vi "ELVIS III v1.1 Open AI (Continuous).vi"(4 "Max Value":dbl[](array[numeric]), 6 "Min Value":dbl[](array[numeric]), 8 "error in (no error)":errorcluster, 10 "Channel Names":string[](array[string]), 11 "Resource name":T7 caption="RIO Device") -> (0 "error out":errorcluster, 1 "Bank Count":u8[](array[numeric]), 2 "AI (Continuous) Channels List":T3 caption="AI Continuous Channels List", 3 "AI (Continuous) Ref Out":T5 caption="AI Continuous Ref Out", 5 "AI (Continous) Read Scale Constants List":T1)   [LabVIEW 2021]
uses:
  <vilib>/userDefined/High Color/nirio_resource_hc.ctl
  <vilib>/myRIO/Common/Instrument Driver Framework/Utilities/typedefs/myRIO v1.0 Reference.ctl
  <vilib>/myRIO/Common/Instrument Driver Framework/Utilities/typedefs/Generic FPGA Reference.ctl
  <vilib>/myRIO/Common/Instrument Driver Framework/ELVIS III v1.0/AI Continuous/typedefs/AI Continuous Channels List.ctl
  <vilib>/myRIO/Common/Instrument Driver Framework/ELVIS III v1.0/AI Continuous/typedefs/ELVIS III v1.0 AI Continuous Channels Enum.ctl
  <vilib>/myRIO/Common/Instrument Driver Framework/Utilities/typedefs/Analog Scaling Constants List.ctl
  <vilib>/myRIO/Common/Instrument Driver Framework/Utilities/typedefs/Analog Scaling Constants.ctl
  <vilib>/myRIO/Common/Instrument Driver Framework/myRIO v1.0/AI Continuous/typedefs/AI Continuous Channels Enum.ctl
  <vilib>/myRIO/Common/Instrument Driver Framework/ELVIS III v1.0/AI Continuous/vis/ELVIS III v1.0 Build MUX Configuration AI Continuous.vi
  <vilib>/Utility/VariantDataType/GetNumericInfo.vi
  <vilib>/myRIO/Common/Instrument Driver Framework/ELVIS III v1.0/Resource Manager/vis/ELVIS III v1.0 Reserve Channel List.vi
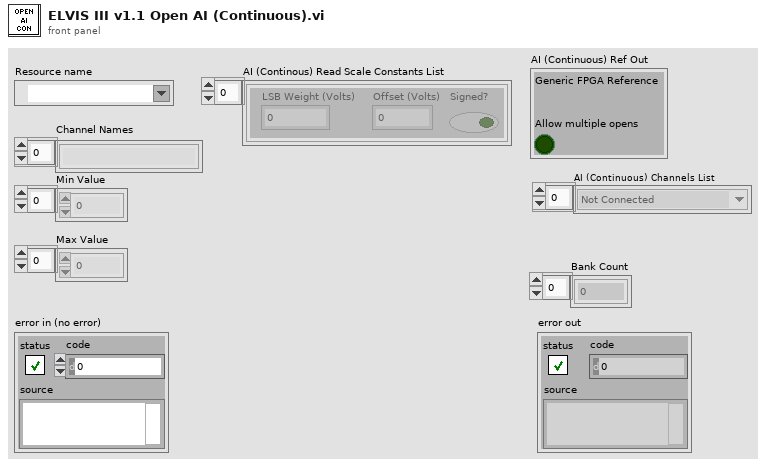
[diagram p1: front panel]
types:
  T1 = typedef "Analog Scaling Constants List.ctl" = T2[]
  T2 = typedef "Analog Scaling Constants.ctl" = cluster{"LSB Weight (Volts)":dbl, "Offset (Volts)":dbl, "Signed?":bool}
  T3 = typedef "AI Continuous Channels List.ctl" = T4[]
  T4 = typedef "ELVIS III v1.0 AI Continuous Channels Enum.ctl" = enum16{"Not Connected", "A/AI0 (Continuous)", "A/AI1 (Continuous)", "A/AI2 (Continuous)", "A/AI3 (Continuous)", "A/AI4 (Continuous)", "A/AI5 (Continuous)", "A/AI6 (Continuous)", "A/AI7 (Continuous)", "A/AI0 (DIFF Continuous)", "A/AI1 (DIFF Continuous)", "A/AI2 (DIFF Continuous)", "A/AI3 (DIFF Continuous)", "B/AI0 (Continuous)", "B/AI1 (Continuous)", "B/AI2 (Continuous)", "B/AI3 (Continuous)", "B/AI4 (Continuous)", "B/AI5 (Continuous)", "B/AI6 (Continuous)", "B/AI7 (Continuous)", "B/AI0 (DIFF Continuous)", "B/AI1 (DIFF Continuous)", "B/AI2 (DIFF Continuous)", "B/AI3 (DIFF Continuous)"}
  T5 = typedef "myRIO v1.0 Reference.ctl" = cluster{"Generic FPGA Reference":T6, "Allow multiple opens":bool}
  T6 = typedef "Generic FPGA Reference.ctl" = refnum<k20>
  T7 = typedef "nirio_resource_hc.ctl" = tag
  T8 = typedef "AI Continuous Channels Enum.ctl" = enum16{"Not Connected", "A/AI0 (Continuous)", "A/AI1 (Continuous)", "A/AI2 (Continuous)", "A/AI3 (Continuous)", "A/AI4 (Continuous)", "A/AI5 (Continuous)", "A/AI6 (Continuous)", "A/AI7 (Continuous)", "A/AI0 (DIFF Continuous)", "A/AI1 (DIFF Continuous)", "A/AI2 (DIFF Continuous)", "A/AI3 (DIFF Continuous)", "B/AI0 (Continuous)", "B/AI1 (Continuous)", "B/AI2 (Continuous)", "B/AI3 (Continuous)", "B/AI4 (Continuous)", "B/AI5 (Continuous)", "B/AI6 (Continuous)", "B/AI7 (Continuous)", "B/AI0 (DIFF Continuous)", "B/AI1 (DIFF Continuous)", "B/AI2 (DIFF Continuous)", "B/AI3 (DIFF Continuous)"}
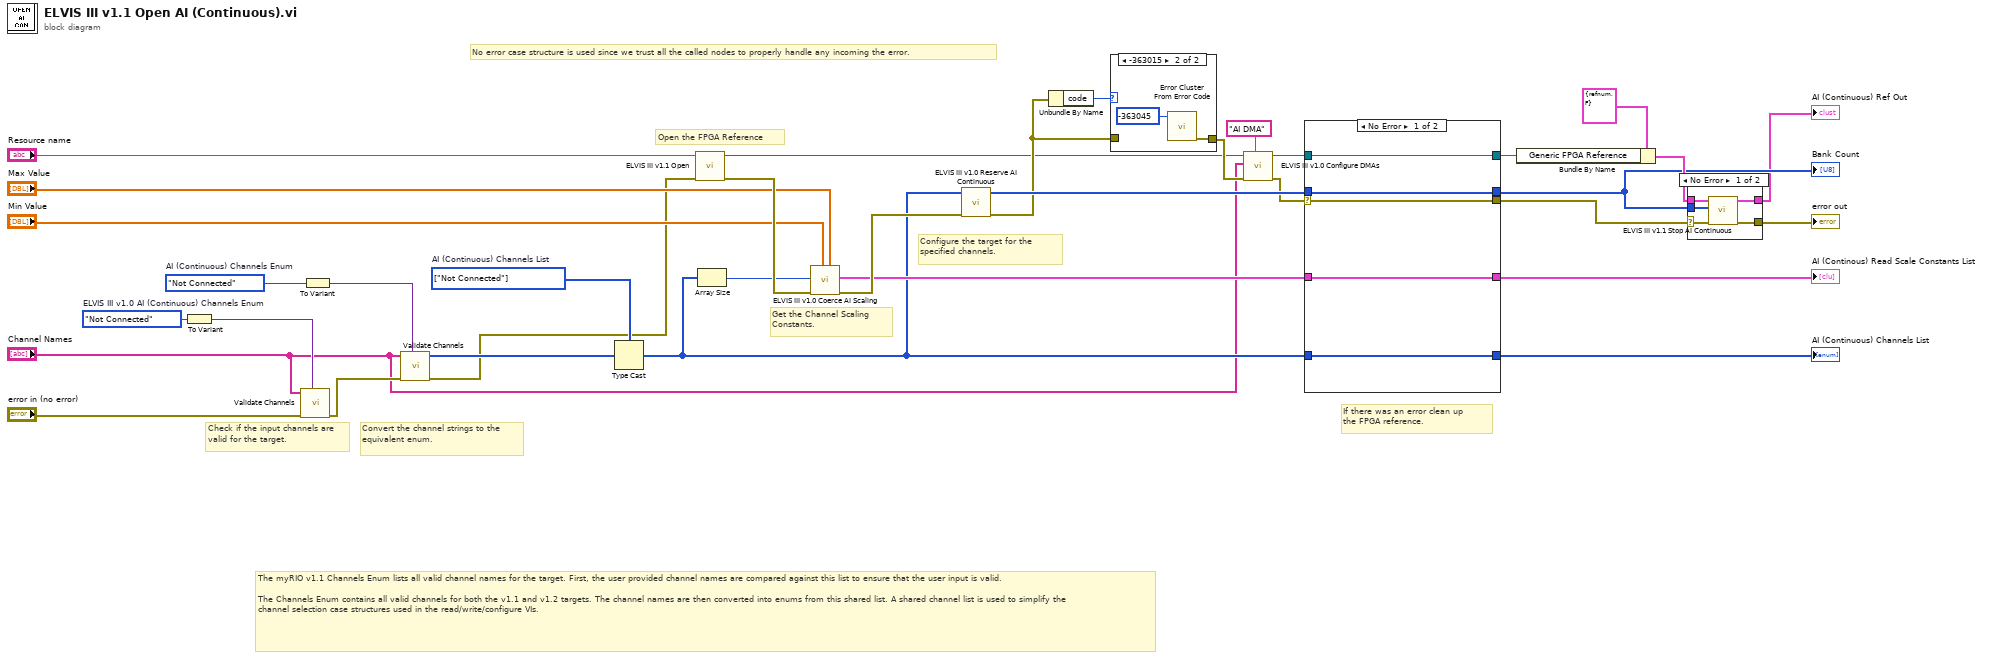
[diagram p0: block diagram]
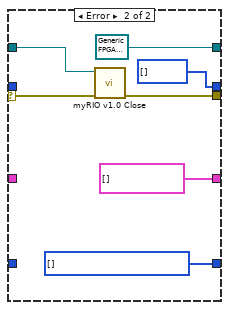
[diagram p4: hidden frame]
diagram:
  w20 = AI_Continuous_Channels_Enum."Not Connected"  # AI (Continuous) Channels Enum
  w25 = T3 [enum."Not Connected"] items=["Not Connected", "A/AI0 (Continuous)", "A/AI1 (Continuous)", "A/AI2 (Continuous)", "A/AI3 (Continuous)", "A/AI4 (Continuous)", "A/AI5 (Continuous)", "A/AI6 (Continuous)", "A/AI7 (Continuous)", "A/AI0 (DIFF Continuous)", "A/AI1 (DIFF Continuous)", "A/AI2 (DIFF Continuous)", "A/AI3 (DIFF Continuous)", "B/AI0 (Continuous)", "B/AI1 (Continuous)", "B/AI2 (Continuous)", "B/AI3 (Continuous)", "B/AI4 (Continuous)", "B/AI5 (Continuous)", "B/AI6 (Continuous)", "B/AI7 (Continuous)", "B/AI0 (DIFF Continuous)", "B/AI1 (DIFF Continuous)", "B/AI2 (DIFF Continuous)", "B/AI3 (DIFF Continuous)"]  # AI (Continuous) Channels List
  w26 = ELVIS_III_v1.0_AI_Continuous_Channels_Enum."Not Connected"  # ELVIS III v1.0 AI (Continuous) Channels Enum
  # "Get the Channel Scaling Constants."
  # "The myRIO v1.1 Channels Enum lists all valid channel names for the target. First, the user provided channel names are compared against this list to ensure that the user input is valid.\n\nThe Channels Enum contains all valid channels for both the v1.1 and v1.2 targets. The channel names are then converted into enums from this shared list. A shared channel list is used to simplify the channel selection case structures used in the read/write/configure VIs."
  # "If there was an error clean up the FPGA reference."
  # "Configure the target for the specified channels."
  # "Open the FPGA Reference"
  # "No error case structure is used since we trust all the called nodes to properly handle any incoming the error."
  # "Convert the channel strings to the equivalent enum."
  # "Check if the input channels are valid for the target."
  n1 = To Variant(anything=w26) -> (Variant=w33:variant)
  n2 = call <vilib>:"Validate Channels.vi"("Channels Enum Variant"=w33, "error in (no error)"="error in (no error)", "Channel Names"="Channel Names") -> ("error out"=w17:errorcluster)  [unwired: 7 in, 1 out]
  n3 = To Variant(anything=w20) -> (Variant=w19:variant)
  n4 = call <vilib>:"Validate Channels.vi"("Channels Enum Variant"=w19, "error in (no error)"=w17, "Channel Names"="Channel Names") -> ("error out"=w16:errorcluster, "Index Array"=w18:u16[])  [unwired: 7 in]
  n5 = Type Cast(type=w25, x=w18) -> (*(type *) &x=w15:T3)
  n6 = call <vilib>:"ELVIS III v1.1 Open.vi"("error in (no error)"=w16, "Resource name"="Resource name") -> ("error out"=w32:errorcluster, "myRIO FPGA Ref Out"=w10:T6)  [unwired: 8 in]
  n7 = Array Size(array=w15) -> (size(s)=w30:i32)
  n8 = call <vilib>:"ELVIS III v1.0 Coerce AI Scaling.vi"("Max Value"="Max Value", "Min Value"="Min Value", "error in (no error)"=w32, "Channel List Size"=w30) -> ("error out"=w31:errorcluster, "Scale Constants Array"=w29:T1)  [unwired: 6 in]
  n9 = call <vilib>:"ELVIS III v1.0 Reserve AI Continuous.vi"("error in (no error)"=w31, "AI (Continuous) Channels List"=w15) -> ("error out"=w12:errorcluster, "Bank Count"=w14:u8[])  [unwired: 8 in]
  n10 = Unbundle By Name(w12) -> ("code"=w13:i32)
  n11 = case shown="-363015" w13 {
    tunnel: w12 -> [w36 _]
    tunnel: [w36 w37] -> w11
    frame Default {
    }
    frame -363015 {
      n12 = call <vilib>:"Error Cluster From Error Code.vi"("error code (0)"=-363045) -> ("error out"=w37:errorcluster)  [unwired: 8 in]
    }
  }
  n13 = call <vilib>:"ELVIS III v1.0 Configure DMAs.vi"("DMA Type"="AI DMA", "error in (no error)"=w11, "Channel Names"="Channel Names", "ELVIS III FPGA Ref"=w10) -> ("error out"=w7:errorcluster, "ELVIS III FPGA Ref"=w8:T6)  [unwired: 6 in]
  n14 = case shown="No Error" w7 {
    selector: w7 -> [w42 w50]
    tunnel: w8 -> [w43 w48]
    tunnel: [w43 T6 refnum ("myRIO FPGA Ref Out")] -> w34
    tunnel: [w42 w49] -> w3
    tunnel: [w41 w45] -> w24
    tunnel: w15 -> [w41 _]
    tunnel: w29 -> [w40 _]
    tunnel: [w40 T1 [] ("AI Block Read Scale Constants List")] -> w23
    tunnel: w14 -> [w39 _]
    tunnel: [w39 u8[] [] ("Bank Count")] -> w4
    frame No Error {
    }
    frame Error {
      w45 = T3 [] items=["Not Connected", "A/AI0 (Continuous)", "A/AI1 (Continuous)", "A/AI2 (Continuous)", "A/AI3 (Continuous)", "A/AI4 (Continuous)", "A/AI5 (Continuous)", "A/AI6 (Continuous)", "A/AI7 (Continuous)", "A/AI0 (DIFF Continuous)", "A/AI1 (DIFF Continuous)", "A/AI2 (DIFF Continuous)", "A/AI3 (DIFF Continuous)", "B/AI0 (Continuous)", "B/AI1 (Continuous)", "B/AI2 (Continuous)", "B/AI3 (Continuous)", "B/AI4 (Continuous)", "B/AI5 (Continuous)", "B/AI6 (Continuous)", "B/AI7 (Continuous)", "B/AI0 (DIFF Continuous)", "B/AI1 (DIFF Continuous)", "B/AI2 (DIFF Continuous)", "B/AI3 (DIFF Continuous)"] ("AI (Continuous) Channels List")
      n15 = call <vilib>:"myRIO v1.0 Close.vi"("error in (no error)"=w50, "myRIO FPGA Ref In"=w48) -> ("error out"=w49:errorcluster)  [unwired: 9 in]
    }
  }
  "AI (Continuous) Channels List" <- w24
  "AI (Continous) Read Scale Constants List" <- w23
  "Bank Count" <- w4
  n16 = Bundle By Name(cluster=T5 {"Generic FPGA Reference"=refnum, "Allow multiple opens"=FALSE} ("myRIO Ref Out"), "Generic FPGA Reference"=w34) -> (w5:T5)
  n17 = case shown="No Error" w3 {
    selector: w3 -> [w53 w57]
    tunnel: w5 -> [w55 w56]
    tunnel: w4 -> [w54 _]
    tunnel: [w52 w57] -> w2
    tunnel: [w51 w56] -> w1
    frame No Error {
      n18 = call <vilib>:"ELVIS III v1.1 Stop AI Continuous.vi"("error in (no error)"=w53, "Bank Count"=w54, "AI (Continuous) Ref In"=w55) -> ("error out"=w52:errorcluster, "AI (Continuous) Ref Out"=w51:T5)  [unwired: 7 in]
    }
    frame Error {
    }
  }
  "error out" <- w2
  "AI (Continuous) Ref Out" <- w1
